vi "Update Display.vi"(8 "error in":errorcluster, 10 "Display Message":string) -> (0 "error out":errorcluster)   [LabVIEW 2024, in "User Interface Control.lvlib"]
uses:
  User Interface Control.lvlib
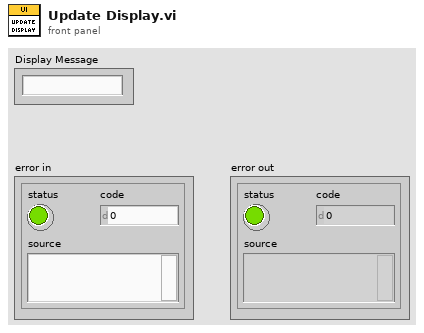
[diagram p1: front panel]
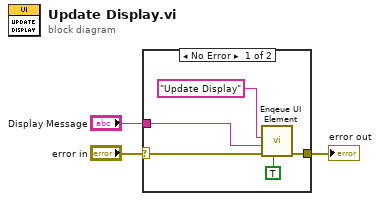
[diagram p0: block diagram]
diagram:
  n1 = case shown="No Error" "error in" {
    selector: "error in" -> [w6 w9]
    tunnel: "Display Message" -> [w7 _]
    tunnel: [w5 w9] -> w2
    frame No Error {
      n2 = call "Enqeue UI Element.vi"("Prioritize Data?"=TRUE, "error in"=w6, "Data"=w7, "Message"="Update Display") -> ("error out"=w5:errorcluster)  [unwired: 7 in]
    }
    frame Error {
    }
  }
  "error out" <- w2
